vi "Teleop.vi"(10 "Match Info":T1={"Autonomous Elapsed Seconds"=0.0, "TeleOp Elapsed Seconds"=0.0, "Disabled Elapsed Seconds"=0.0, "Visited Autonomous"=FALSE, "Visited TeleOp"=FALSE, "Visited Disabled"=FALSE, "Autonomous Settings"={"Autonomous Style"=enum."Independent", "VI Refnum"=refnum}}, 11 "Call Context":T2) -> ()   [LabVIEW 2014]
doc: "This VI is called for each TeleOp packet received from the DS where the robot is not disabled. It is often used to read from the joysticks and update I/O or to update setpoints for timed control loops. It should complete and return within 20 milliseconds or it may miss DS packets."
uses:
  <vilib>/Rock Robotics/WPI/DriverStation/WPI_DriverStationDerivedRobotMode.ctl
  <vilib>/Rock Robotics/WPI/DriverStation/WPI_DriverStationMatch Info.ctl
  <vilib>/Rock Robotics/WPI/Solenoid/WPI_SolenoidValue.ctl
  <vilib>/Rock Robotics/WPI/Relay/WPI_RelayValue.ctl
  <vilib>/Rock Robotics/WPI/RobotDrive/WPI_RobotDriveGetSetRefNum.vi
  <vilib>/Rock Robotics/WPI/Joystick/WPI_JoystickGetSetRefNum.vi
  Robot Global Data.vi
  <vilib>/Rock Robotics/WPI/Solenoid/WPI_SolenoidSetEnum.vi
panel:
  out "toggle on/off":bool=TRUE
  in  "toggle on/off internal":bool=TRUE
  in  "last switch":bool
  out "Numeric 1":dbl(slide) scale=0.0..100.0
  out "Boolean 2":bool
  out "Boolean 1":bool
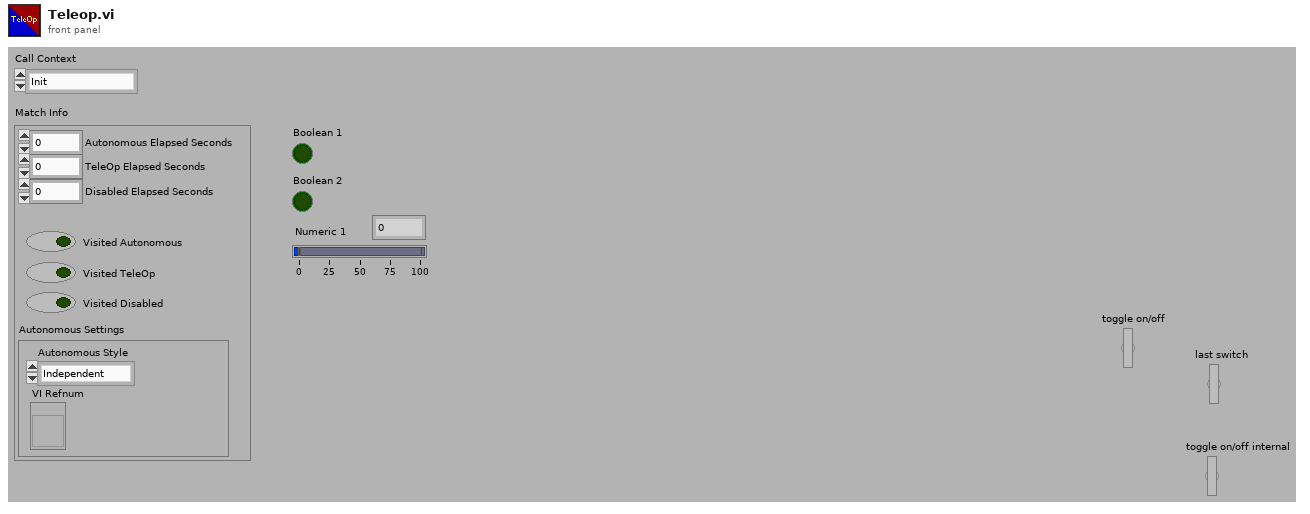
[diagram p1: front panel]
types:
  T1 = typedef "WPI_DriverStationMatch Info.ctl" = cluster{"Autonomous Elapsed Seconds":dbl, "TeleOp Elapsed Seconds":dbl, "Disabled Elapsed Seconds":dbl, "Visited Autonomous":bool, "Visited TeleOp":bool, "Visited Disabled":bool, "Autonomous Settings":cluster{"Autonomous Style":enum16{"Iterative", "Independent"}, "VI Refnum":refnum<vi>}}
  T2 = typedef "WPI_DriverStationDerivedRobotMode.ctl" = enum16{"Init", "Execute", "Stop"}
  T3 = typedef "WPI_RelayValue.ctl" = enum16{"Off", "On", "Forward", "Reverse"}
  T4 = typedef "WPI_SolenoidValue.ctl" = enum16{"Off", "On", "Forward", "Reverse"}
  T5 = typedef "WPI_RobotDriveDevRef.ctl" = cluster{"DevStatus":errorcluster, "Motors[]":T6[], "Square Inputs":bool, "Max Output":dbl}
  T6 = typedef "WPI_MotorControlDeviceRef.ctl" = cluster{"DeviceStatus":errorcluster, "Type":enum16{"PWM", "CAN"}, "PWM":cluster{"Digital Module":T7, "PWM Channel":T8, "DeadBand":T9}, "CAN":cluster{"Device Number":u8, "Control Mode":T10, "Semaphore":T11, "Max Vout":dbl}, "Invert":bool, "TransformRef":T12, "InvTransformRef":T12}
  T7 = typedef "FPGA_TypedefDigitalModule.ctl" = enum16{"Digital Module 1", "Digital Module 2"}
  T8 = typedef "FPGA_DIOPWMChannel.ctl" = enum8{"PWM 1", "PWM 2", "PWM 3", "PWM 4", "PWM 5", "PWM 6", "PWM 7", "PWM 8", "PWM 9", "PWM 10", "Invalid"}
  T9 = typedef "WPI_PWMDeadband.ctl" = cluster{"Name":string, "maxPositivePwm":i32, "minPositivePwm":i32, "centerPwm":i32, "maxNegativePwm":i32, "minNegativePwm":i32, "angularRange":u16}
  T10 = typedef "WPI_CANJaguar_ControlMode.ctl" = enum8{"Percent VBus", "Current", "Speed", "Position", "Voltage"}
  T11 = typedef "Semaphore RefNum" = refnum<k1>
  T12 = typedef "WPI_PWMTransform_ConPane.ctl" = refnum<vi>
  T13 = typedef "WPI_JoystickDevRef.ctl" = cluster{"Device":T14}
  T14 = typedef "WPI_JoystickDeviceEnum.ctl" = enum16{"USB 0", "USB 1", "USB 2", "USB 3", "USB 4", "USB 5"}
  T15 = cluster{"Button 1":bool, "Button 2":bool, "Button 3":bool, "Button 4":bool, "Button 5":bool, "Button 6":bool, "Button 7":bool, "Button 8":bool, "Button 9":bool, "Button 10":bool, "Button 11":bool, "Button 12":bool}
  T16 = cluster{"axis 1 (x)":dbl, "axis 2 (y)":dbl, "axis 3 (throttle)":dbl, "axis 4":dbl, "axis 5":dbl, "axis 6":dbl}
  T17 = typedef "WPI_SolenoidDevRef.ctl" = cluster{"DevStatus":errorcluster, "Solenoid Module":T18, "Forward Solenoid Channel":T19, "Reverse Solenoid Channel":T19}
  T18 = typedef "FPGA_TypedefSolenoidModule.ctl" = enum16{"Solenoid Module 1", "Solenoid Module 2"}
  T19 = typedef "WPI_SolenoidChannel.ctl" = enum8{"Solenoid 1", "Solenoid 2", "Solenoid 3", "Solenoid 4", "Solenoid 5", "Solenoid 6", "Solenoid 7", "Solenoid 8", "Invalid"}
  T20 = typedef "WPI_RelayDevRef.ctl" = cluster{"DevStatus":errorcluster, "Relay Channel":T21, "Digital Module":T7, "Relay Direction":T22}
  T21 = typedef "FPGA_DIORelayChannel.ctl" = enum8{"Relay 1", "Relay 2", "Relay 3", "Relay 4", "Relay 5", "Relay 6", "Relay 7", "Relay 8", "Invalid"}
  T22 = typedef "WPI_RelayDirection.ctl" = enum16{"Both directions", "Forward only", "Reverse only"}
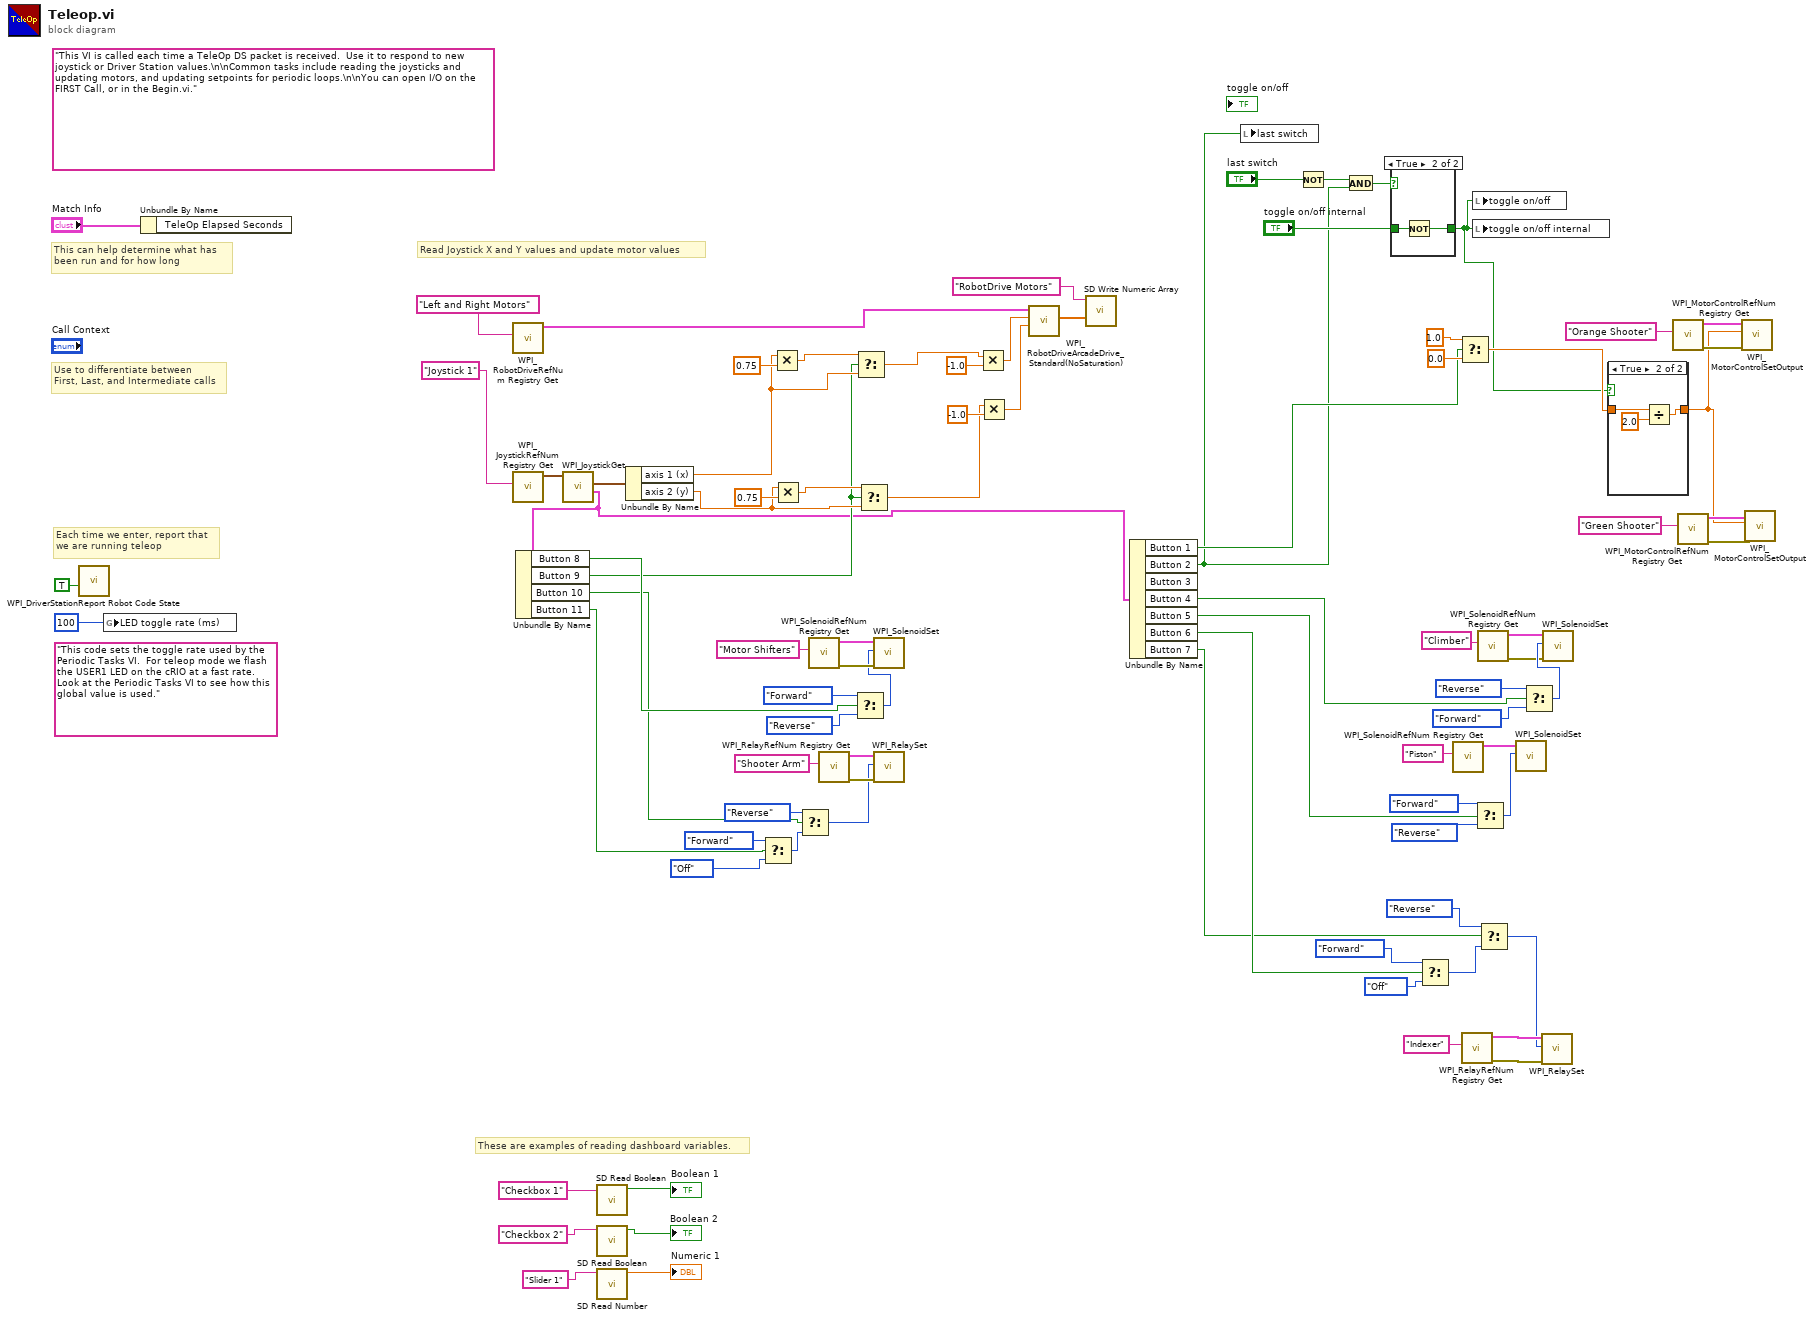
[diagram p0: block diagram]
diagram:
  (unwired) "This code sets the toggle rate used by the Periodic Tasks VI.  For teleop mode we flash the USER1 LED on the cRIO at a fast rate.  Look at the Periodic Tasks VI to see how this global value is used."
  (unwired) "This VI is called each time a TeleOp DS packet is received.  Use it to respond to new joystick or Driver Station values.\n\nCommon tasks include reading the joysticks and updating motors, and updating setpoints for periodic loops.\n\nYou can open I/O on the FIRST Call, or in the Begin.vi."
  # "These are examples of reading dashboard variables."
  # "Each time we enter, report that\nwe are running teleop"
  # "Use to differentiate between\nFirst, Last, and Intermediate calls"
  # "This can help determine what has\nbeen run and for how long"
  # "Read Joystick X and Y values and update motor values"
  n1 = call <vilib>:"WPI_DriverStationReport Robot Code State.vi"("TeleOp"=TRUE ("Autonomous")) -> ()  [unwired: 10 in, 1 out]
  n2 = global write "Robot Global Data.vi" "LED toggle rate (ms)"(u32 100 ("LED ms toggle rate")) -> ()
  n3 = Unbundle By Name("Match Info") -> ()  [unwired: 1 out]
  n4 = call <vilib>:"WPI_RobotDriveRefNum Registry Get.vi"("refnum name"="Left and Right Motors") -> ("RobotDriveDevRef"=w85:T5)  [unwired: 1 in, 9 out]
  n5 = call <vilib>:"WPI_JoystickRefNum Registry Get.vi"("refnum name"="Joystick 1") -> ("JoystickDevRef"=w83:T13)  [unwired: 1 in, 9 out]
  n6 = call <vilib>:"WPI_JoystickGet.vi"("JoystickDevRef"=w83) -> ("Buttons"=w15:T15, "Axes"=w80:T16)  [unwired: 1 in, 4 out]
  n7 = Unbundle By Name(w15) -> ("Button 8"=w37:bool, "Button 9"=w30:bool, "Button 10"=w17:bool, "Button 11"=w16:bool)
  n8 = call <vilib>:"SD Read Boolean.vi"("Name"="Checkbox 1" ("refnum name")) -> ("Boolean"=→"Boolean 1":bool)  [unwired: 8 in, 2 out]
  n9 = call <vilib>:"SD Read Boolean.vi"("Name"="Checkbox 2" ("refnum name")) -> ("Boolean"=→"Boolean 2":bool)  [unwired: 8 in, 2 out]
  n10 = call <vilib>:"SD Read Number.vi"("Name"="Slider 1" ("refnum name")) -> ("Numeric"=→"Numeric 1":dbl)  [unwired: 8 in, 2 out]
  n11 = Unbundle By Name(w80) -> ("axis 1 (x)"=w32:dbl, "axis 2 (y)"=w31:dbl)
  n12 = Select(t=WPI_SolenoidValue."Forward" ("Value"), s=w16, f=WPI_RelayValue."Off" ("RelayValue")) -> (s? t:f=w50:T3)
  n13 = Multiply(x=w32, y=0.75) -> (x*y=w35:dbl)
  n14 = Multiply(x=w31, y=0.75) -> (x*y=w36:dbl)
  n15 = Select(t=WPI_SolenoidValue."Reverse" ("Value"), s=w17, f=w50) -> (s? t:f=w49:T3)
  n16 = call <vilib>:"WPI_SolenoidRefNum Registry Get.vi"("refnum name"="Motor Shifters") -> ("error out"=w71:errorcluster, "SolenoidDevRef"=w70:T17)  [unwired: 9 in]
  n17 = call <vilib>:"WPI_RelayRefNum Registry Get.vi"("refnum name"="Shooter Arm") -> ("error out"=w58:errorcluster, "RelayDevRef"=w55:T20)  [unwired: 9 in]
  n18 = Select(t=WPI_SolenoidValue."Forward" ("Value"), s=w37, f=WPI_SolenoidValue."Reverse" ("Value")) -> (s? t:f=w66:T4)
  n19 = Select(t=w35, s=w30, f=w32) -> (s? t:f=w9:dbl)
  n20 = Select(t=w36, s=w30, f=w31) -> (s? t:f=w12:dbl)
  n21 = call-poly <vilib>:"WPI_SolenoidSet.vi"("error in (no error)"=w71, "Value"=w66, "SolenoidDevRef"=w70) -> ()  [unwired: 7 in, 2 out]
  n22 = call <vilib>:"WPI_RelaySet.vi"("error in (no error)"=w58, "RelayValue"=w49, "RelayDevRef"=w55) -> ()  [unwired: 7 in, 2 out]
  n23 = Multiply(x=w9, y=-1.0) -> (x*y=w10:dbl)
  n24 = Multiply(x=w12, y=-1.0) -> (x*y=w11:dbl)
  n25 = call <vilib>:"WPI_RobotDriveArcadeDrive_Standard(NoSaturation).vi"("Y axis value"=w11, "X axis value"=w10, "RobotDriveDevRef"=w85) -> ("Motor Values"=w78:dbl[])  [unwired: 1 in, 7 out]
  n26 = call <vilib>:"SD Write Numeric Array.vi"("Numeric Array"=w78, "Name"="RobotDrive Motors") -> ()  [unwired: 8 in, 2 out]
  n27 = Unbundle By Name(w15) -> ("Button 1"=w7:bool, "Button 2"=w1:bool, "Button 4"=w19:bool, "Button 5"=w29:bool, "Button 6"=w24:bool, "Button 7"=w20:bool)  [unwired: 1 out]
  n28 = local write "last switch"(w1) -> ()
  n29 = Not(x="last switch") -> (.not. x?=w5:bool)
  n30 = And(x=w5, y=w1) -> (x .and. y?=w4:bool)
  n31 = case shown="True" w4 {
    tunnel: "toggle on/off internal" -> [w88 w90]
    tunnel: [w88 w89] -> w2
    frame False {
    }
    frame True {
      n32 = Not(x=w90) -> (.not. x?=w89:bool)
    }
  }
  n33 = Select(t=WPI_RelayValue."Forward" ("RelayValue"), s=w24, f=WPI_RelayValue."Off" ("RelayValue")) -> (s? t:f=w23:T3)
  n34 = call <vilib>:"WPI_SolenoidRefNum Registry Get.vi"("refnum name"="Piston") -> ("SolenoidDevRef"=w48:T17)  [unwired: 9 in, 1 out]
  n35 = Select(t=1.0, s=w7, f=0.0) -> (s? t:f=w18:dbl)
  n36 = call <vilib>:"WPI_RelayRefNum Registry Get.vi"("refnum name"="Indexer") -> ("error out"=w56:errorcluster, "RelayDevRef"=w57:T20)  [unwired: 9 in]
  n37 = local write "toggle on/off"(w2) -> ()
  n38 = local write "toggle on/off internal"(w2) -> ()
  n39 = Select(t=WPI_SolenoidValue."Forward" ("Value"), s=w29, f=WPI_SolenoidValue."Reverse" ("Value")) -> (s? t:f=w44:T4)
  n40 = call <vilib>:"WPI_SolenoidRefNum Registry Get.vi"("refnum name"="Climber") -> ("error out"=w38:errorcluster, "SolenoidDevRef"=w39:T17)  [unwired: 9 in]
  n41 = Select(t=WPI_RelayValue."Reverse" ("RelayValue"), s=w20, f=w23) -> (s? t:f=w21:T3)
  n42 = call-poly <vilib>:"WPI_SolenoidSet.vi"("Value"=w44, "SolenoidDevRef"=w48) -> ()  [unwired: 8 in, 2 out]
  n43 = Select(t=WPI_SolenoidValue."Reverse" ("Value"), s=w19, f=WPI_SolenoidValue."Forward" ("Value")) -> (s? t:f=w43:T4)
  n44 = call <vilib>:"WPI_RelaySet.vi"("error in (no error)"=w56, "RelayValue"=w21, "RelayDevRef"=w57) -> ()  [unwired: 7 in, 2 out]
  n45 = call-poly <vilib>:"WPI_SolenoidSet.vi"("error in (no error)"=w38, "Value"=w43, "SolenoidDevRef"=w39) -> ()  [unwired: 7 in, 2 out]
  n46 = case shown="True" w2 {
    tunnel: [w91 w92] -> w8
    tunnel: w18 -> [w91 w94]
    frame False {
    }
    frame True {
      n47 = Divide(x=w94, y=2.0) -> (x/y=w92:dbl)
    }
  }
  n48 = call <vilib>:"WPI_MotorControlRefNum Registry Get.vi"("refnum name"="Orange Shooter") -> ("error out"=w61:errorcluster, "MotorControlDevRef"=w60:T6)  [unwired: 9 in]
  n49 = call <vilib>:"WPI_MotorControlRefNum Registry Get.vi"("refnum name"="Green Shooter") -> ("error out"=w62:errorcluster, "MotorControlDevRef"=w63:T6)  [unwired: 9 in]
  n50 = call <vilib>:"WPI_MotorControlSetOutput.vi"("error in (no error)"=w61, "Output"=w8, "MotorControlDevRef"=w60) -> ()  [unwired: 6 in, 3 out]
  n51 = call <vilib>:"WPI_MotorControlSetOutput.vi"("error in (no error)"=w62, "Output"=w8, "MotorControlDevRef"=w63) -> ()  [unwired: 6 in, 3 out]
